vi "Init from Element.vi"(8 "error in (no error)":errorcluster, 10 "Config Element":refnum<class "Config Element.lvclass">, 11 "Seq Element in":refnum<class "Seq Element.lvclass">) -> (0 "error out":errorcluster, 3 "Seq Element out":refnum<class "Seq Element.lvclass">)   [LabVIEW 2020, in "Seq Element.lvclass"]
uses:
  Seq Element.lvclass
  lv-cdm/CDM-Config/Config Element/Config Element.lvclass
  Seq Element.lvclass/Seq Element.ctl
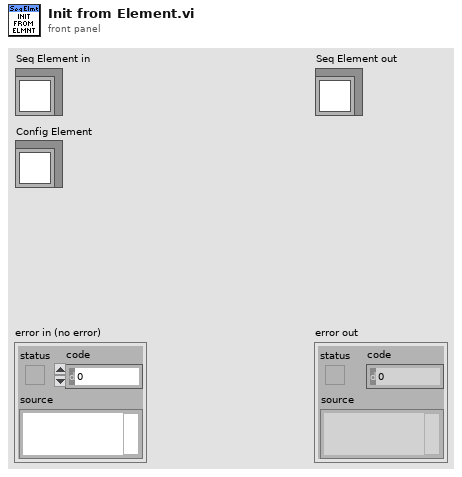
[diagram p1: front panel]
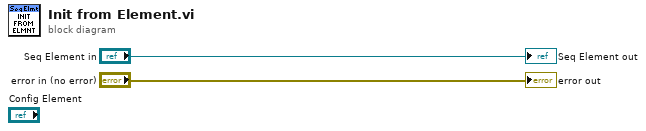
[diagram p0: block diagram]
diagram:
  "error out" <- "error in (no error)"
  "Seq Element out" <- "Seq Element in"
